vi "gyroTurn.vi"(11 "Angle":dbl) -> ()   [LabVIEW 2015]
uses:
  Robot Global Data.vi
  <vilib>/addons/control/pid/pid.llb/PID (DBL).vi
  <vilib>/addons/control/pid/NI_PID_pid.lvlib
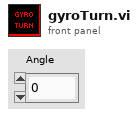
[diagram p1: front panel]
types:
  T1 = typedef "WPI_GyroDevRef.ctl" = cluster{"DevStatus":errorcluster, "Analog Channel":T2, "Offset":dbl, "Gain (VoltsPerDegree/Second)":dbl, "Gyro Type":enum16{"Analog", "XRS450"}, "Handle":i32, "SPI Bus":T3, "Device Found":bool, "Sample Rate":dbl, "Calibrate On Open":bool}
  T2 = typedef "FPGA_AIChannel.ctl" = enum8{"AI 0", "AI 1", "AI 2", "AI 3", "AI MXP 0", "AI MXP 1", "AI MXP 2", "AI MXP 3", "Invalid"}
  T3 = typedef "spi_bus.ctl" = enum16{"SPI On-Board, CS0", "SPI On-Board, CS1", "SPI On-Board, CS2", "SPI On-Board, CS3", "SPI MXP", "Invalid"}
  T4 = cluster{"proportional gain (Kc)":dbl, "integral time (Ti, min)":dbl, "derivative time (Td, min)":dbl}
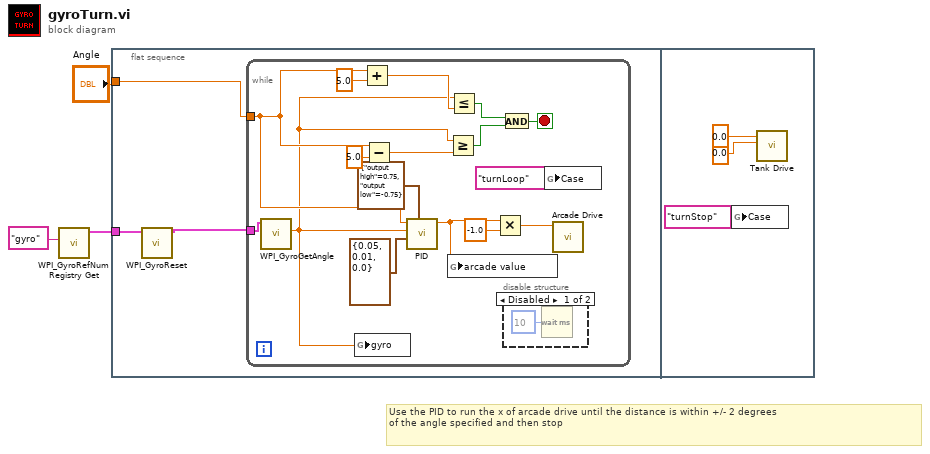
[diagram p0: block diagram]
diagram:
  # "Use the PID to run the x of arcade drive until the distance is within +/- 2 degrees\nof the angle specified and then stop"
  n1 = call <vilib>:"WPI_GyroRefNum Registry Get.vi"("refnum name"="gyro") -> ("GyroDevRef"=w2:T1)  [unwired: 9 in, 1 out]
  n2 = flat-sequence {
    tunnel: w2 -> [w5]
    tunnel: "Angle" -> [w4]
    frame #0 {
      n3 = call <vilib>:"WPI_GyroReset.vi"("GyroDevRef"=w5) -> ("GyroDevRef"=w6:T1)  [unwired: 9 in, 1 out]
      n4 = while {
        tunnel: w6 -> [w22]
        tunnel: w4 -> [w15]
        stop <- w14 stop-if-true
        n5 = call <vilib>:"WPI_GyroGetAngle.vi"("GyroDevRef"=w22) -> ("Angle"=w10:dbl)  [unwired: 6 in, 4 out]
        n6 = global write "Robot Global Data.vi" "gyro"(w10) -> ()
        n7 = Add(x=w15, y=5.0) -> (x+y=w16:dbl)
        n8 = Subtract(x=w15, y=5.0) -> (x-y=w17:dbl)
        n9 = call-poly <vilib>:"PID.vi"("output range"=cluster{"output high":dbl, "output low":dbl} {"output high"=0.75, "output low"=-0.75}, "PID gains"=T4 {"proportional gain (Kc)"=0.05, "integral time (Ti, min)"=0.01, "derivative time (Td, min)"=0.0}, "process variable"=w10, "setpoint"=w15) -> ("output"=w9:dbl)  [unwired: 6 in, 1 out]
        n10 = Greater Or Equal?(x=w10, y=w17) -> (x >= y?=w12:bool)
        n11 = global write "Robot Global Data.vi" "arcade value"(w9) -> ()
        n12 = Less Or Equal?(x=w10, y=w16) -> (x <= y?=w13:bool)
        n13 = Multiply(x=w9, y=-1.0) -> (x*y=w8:dbl)
        n14 = And(x=w13, y=w12) -> (x .and. y?=w14:bool)
        n15 = disable-structure shown="Disabled" {
          frame Disabled {
            n16 = Wait (ms)(milliseconds to wait=u32 10) -> ()  [unwired: 1 out]
          }
          frame Enabled {
          }
        }
        n17 = global write "Robot Global Data.vi" "Case"("turnLoop" ("Case")) -> ()
        n18 = call "Arcade Drive.vi"("x"=w8) -> ()  [unwired: 11 in]
      }
    }
    frame #1 {
      n19 = global write "Robot Global Data.vi" "Case"("turnStop" ("Case")) -> ()
      n20 = call "Tank Drive.vi"("Right"=0.0 ("y"), "Left"=0.0 ("x")) -> ()  [unwired: 10 in]
    }
  }
